vi "Clear Path.vi"(8 "error in (no error)":errorcluster, 11 "Reference Control in":refnum<class "Reference Control.lvclass">) -> (0 "error out":errorcluster, 3 "Reference Control out":refnum<class "Reference Control.lvclass">)   [LabVIEW 2016, in "Reference Control.lvclass"]
uses:
  Reference Control.lvclass
  Reference Control.lvclass/Reference Control.ctl
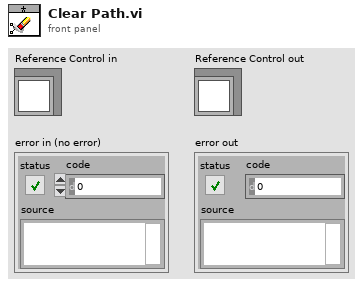
[diagram p1: front panel]
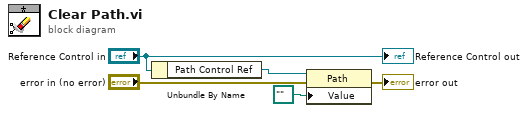
[diagram p0: block diagram]
diagram:
  n1 = Unbundle By Name("Reference Control in") -> ("Path Control Ref"=w1:refnum<vi>)
  n2 = property class="Path"(reference=w1, error in="error in (no error)", "Value"=path "" ("Path")) -> (error out=→"error out":errorcluster)  [unwired: 1 out]
  "Reference Control out" <- "Reference Control in"
